vi "Trigger Slope.vi"(7 "Read Value? (F)":bool, 8 "error in (no error)":errorcluster, 10 "Trigger Slope (Rise)":T1, 11 "VISA resource name":refnum<visa-resource-name>) -> (0 "error out":errorcluster, 2 "Trigger Slope":T1, 3 "VISA resource name out":refnum<visa-resource-name>)   [LabVIEW 2013, in "SRS SR400.lvlib"]
doc: "<B>TS { j }</B>\n\nIf j = 1, the TS command sets the gate trigger slope to FALL or negative. If j = 0, the gate trigger slope is set to RISE or positive. If j is absent, the gate trigger slope is returned."
uses:
  <instrlib>/SRS SR400/SRS SR400.lvlib
  <instrlib>/SRS SR400/Public/Typedefs/Trigger Slope.ctl
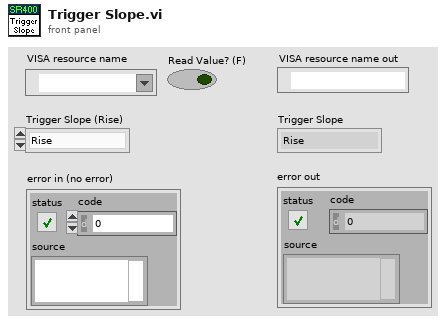
[diagram p1: front panel]
types:
  T1 = typedef "SRS SR400.lvlib/Trigger Slope.ctl" = enum16{"Rise", "Fall"}
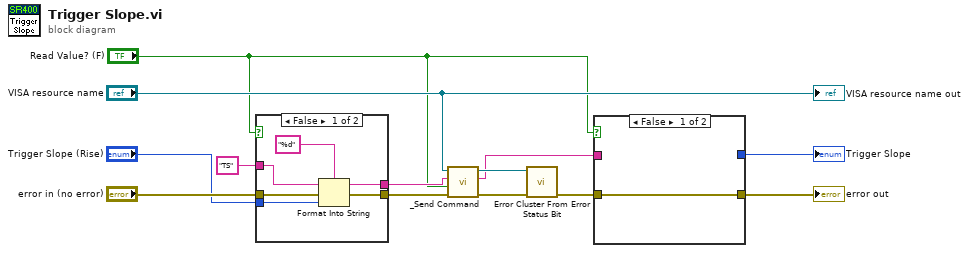
[diagram p0: block diagram]
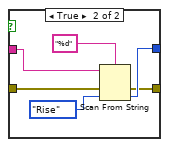
[diagram p2: hidden frame]
diagram:
  n1 = case shown="False" "Read Value? (F)" {
    tunnel: "error in (no error)" -> [w19 w20]
    tunnel: [w17 w21] -> w12
    tunnel: [w16 w20] -> w11
    tunnel: "Trigger Slope (Rise)" -> [w15 _]
    tunnel: "TS" ("command") -> [w14 w21]
    frame False {
      n2 = Format Into String(format string="%d", initial string=w14, error in=w19, w15) -> (resulting string=w17:string, error out=w16:errorcluster)
    }
    frame True {
    }
  }
  n3 = call <instrlib>:"_Send Command.vi"("error in (no error)"=w11, "Read Value? (F)"="Read Value? (F)", "Command"=w12, "VISA resource name"="VISA resource name") -> ("error out"=w7:errorcluster, "Response"=w4:string, "VISA resource name out"=w8:refnum<visa-resource-name>)  [unwired: 5 out]
  n4 = call <instrlib>:"Error Cluster From Error Status Bit.vi"("error in (no error)"=w7, "VISA resource name"=w8) -> ("error out"=w5:errorcluster)  [unwired: 8 in, 1 out]
  n5 = case shown="False" "Read Value? (F)" {
    tunnel: w5 -> [w22 w28]
    tunnel: w4 -> [_ w25]
    tunnel: [_ w24] -> w3
    tunnel: [w22 w23] -> w2
    frame False {
    }
    frame True {
      n6 = Scan From String(format string="%d", input string=w25, error in=w28, default 1=Trigger_Slope."Rise" ("Slope")) -> (error out=w23:errorcluster, output 1=w24:T1)  [unwired: 1 in, 2 out]
    }
  }
  "error out" <- w2
  "Trigger Slope" <- w3
  "VISA resource name out" <- "VISA resource name"
